vi "JPARC_foil_I_monitor.vi"() -> ()   [LabVIEW 2017]
uses:
  <instrlib>/Agilent 34401/Agilent 34401.lvlib
panel:
  out "Graph (I)":cluster{timestamp[], dbl[]}(graph)={[timestamp(3708901329.025436 s since 1904-01-01), timestamp(3708901330.0249934 s since 1904-01-01), timestamp(3708901331.0253873 s since 1904-01-01), timestamp(3708901332.024697 s since 1904-01-01), timestamp(3708901333.024849 s since 1904-01-01), timestamp(3708901334.026148 s since 1904-01-01), timestamp(3708901335.027178 s since 1904-01-01), timestamp(3708901336.028392 s since 1904-01-01), timestamp(3708901337.029397 s since 1904-01-01), timestamp(3708901338.0297656 s since 1904-01-01), timestamp(3708901339.030303 s since 1904-01-01), timestamp(3708901340.0303473 s since 1904-01-01), timestamp(3708901341.0305457 s since 1904-01-01), timestamp(3708901342.0300026 s since 1904-01-01), timestamp(3708901343.0298033 s since 1904-01-01), timestamp(3708901344.031312 s since 1904-01-01), timestamp(3708901345.030869 s since 1904-01-01), timestamp(3708901346.031209 s since 1904-01-01), timestamp(3708901347.0307384 s since 1904-01-01), timestamp(3708901348.030896 s since 1904-01-01), timestamp(3708901349.032491 s since 1904-01-01), timestamp(3708901350.0335054 s since 1904-01-01), timestamp(3708901351.0332375 s since 1904-01-01), timestamp(3708901352.0330696 s since 1904-01-01), timestamp(3708901353.032852 s since 1904-01-01)], [-4.97e-08, -2.9e-08, -1.015e-07, -7.04e-08, 1.45e-08, -1.036e-07, 1.66e-08, -1.574e-07, -1.678e-07, -4.35e-08, -1.325e-07, -1.367e-07, -1.408e-07, -1.036e-07, -1.325e-07, -1.47e-07, -1.346e-07, -3.73e-08, -7.87e-08, -1.781e-07, -9.11e-08, -1.408e-07, -1.16e-07, -1.056e-07, -1.201e-07]} caption="XY Graph"
  in  "stop":bool
  in  "COMMENT":string="_I_monitor"
  in  "base path":path=path "C:/LabVIEW/DATA/J-PARC_202107/test_0712"
  in  "wait (s)":dbl=1.0 format="%#_13g"
  out "Measurement":dbl=-1.201e-07
  out "error out":errorcluster
  in  "VISA resource name":refnum<visa-resource-name>="GPIB0::19::INSTR"
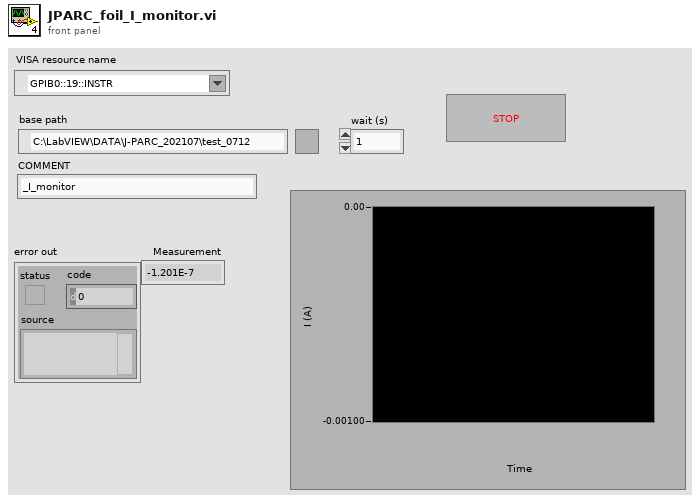
[diagram p1: front panel]
types:
  T1 = enum16{"open", "replace", "create", "open or create", "replace or create", "replace or create with confirmation"}
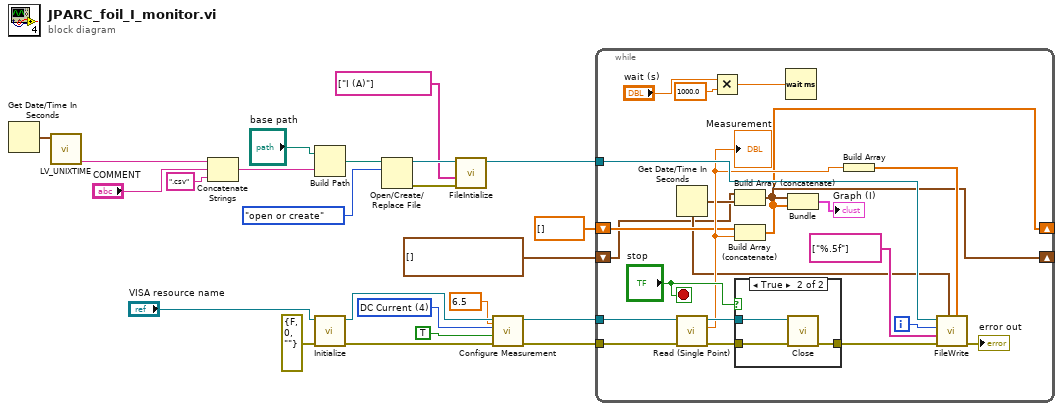
[diagram p0: block diagram]
diagram:
  w2 = u16 4 items=["DC Voltage", "AC Voltage", "2 - Wire Resistance", "4 - Wire Resistance", "DC Current", "AC Current", "Frequency", "Period", "Continuity", "Diode Checking", "VDC:VDC Ratio", "Temperature", "Capacitance"] ("Function (0: DC Voltage)")
  w3 = 6.5 items=["4.5"=4.5, "5.5"=5.5, "6.5"=6.5] ("Manual Resolution (5.5 Digits)")
  n1 = Get Date/Time In Seconds() -> (seconds since 1Jan1904=w20:timestamp)
  n2 = call "LV_UNIXTIME.vi"("current time"=w20) -> ("date/time string"=w11:string)  [unwired: 9 in, 1 out]
  n3 = Concatenate Strings(w11, "COMMENT", ".csv" ("string")) -> (w17:string)
  n4 = Build Path(base path="base path", name or relative path=w17) -> (appended path=w19:path)
  n5 = call "Initialize.vi"("error in (no error)"=errorcluster {"status"=FALSE, "code"=0, "source"=""}, "VISA resource name"="VISA resource name") -> ("error out"=w7:errorcluster, "VISA resource name out"=w4:refnum<visa-resource-name>)  [unwired: 8 in]
  n6 = Open/Create/Replace File(file path (use dialog)=w19, operation (0:open)=T1."open or create") -> (refnum out=w14:refnum<file>, error out=w15:errorcluster)  [unwired: 4 in, 1 out]
  n7 = call "FileIntialize.vi"("Error In"=w15, "Labels"=string[] ["I (A)"], "refnum in"=w14) -> ("File Refnum"=w10:refnum<file>)  [unwired: 7 in, 1 out]
  n8 = call <instrlib>:"Configure Measurement.vi"("Manual Resolution (5.5 Digits)"=w3, "error in (no error)"=w7, "Enable Auto Range (T: Enable)"=TRUE, "Function (0: DC Voltage)"=w2, "VISA resource name"=w4) -> ("error out"=w6:errorcluster, "VISA resource name out"=w5:refnum<visa-resource-name>)  [unwired: 5 in]
  n9 = while {
    tunnel: w5 -> [w44]
    tunnel: w6 -> [w43]
    tunnel: w10 -> [w36]
    shift-right: [w25] -> _
    shift-left: dbl[] [] -> [w29]
    shift-right: [w26] -> _
    shift-left: timestamp[] [] -> [w27]
    i -> [w35]
    stop <- "stop" stop-if-true
    n10 = Get Date/Time In Seconds() -> (seconds since 1Jan1904=w28:timestamp)
    n11 = call "Read (Single Point).vi"("error in (no error)"=w43, "VISA resource name"=w44) -> ("error out"=w37:errorcluster, "Measurement"=w30:dbl, "VISA resource name out"=w38:refnum<visa-resource-name>)  [unwired: 7 in]
    "Measurement" <- w30
    n12 = Multiply(x="wait (s)", y=1000.0 ("Measurement 2")) -> (x*y=w42:dbl)
    n13 = Build Array (concatenate)(w27, w28) -> (w26:timestamp[])
    n14 = Build Array (concatenate)(w29, w30) -> (w25:dbl[])
    n15 = case shown="True" "stop" {
      tunnel: w38 -> [_ w48]
      tunnel: [w45 w47] -> w33
      tunnel: w37 -> [w45 w46]
      frame False {
      }
      frame True {
        n16 = call <instrlib>:"Close.vi"("error in (no error)"=w46, "VISA resource name"=w48) -> ("error out"=w47:errorcluster)  [unwired: 9 in]
      }
    }
    n17 = Wait (ms)(milliseconds to wait=w42) -> ()  [unwired: 1 out]
    n18 = Bundle(w26, w25) -> (→"Graph (I)":cluster{timestamp[], dbl[]})  [unwired: 1 in]
    n19 = Build Array(w30) -> (w31:dbl[])
    n20 = call "FileWrite.vi"("DataArray"=w31, "Time Stamp"=w28, "Error In"=w33, "FileFormat"=string[] ["%.5f"], "Index"=w35, "refnum in"=w36) -> ("Error Out"=→"error out":errorcluster)  [unwired: 4 in, 1 out]
  }
